vi "getTaskReference.vi"(8 "error in (no error)":errorcluster, 11 "ITaskClassTemplate in":refnum<class "ITaskClassTemplate.lvclass">) -> (0 "error out":errorcluster, 2 "taskRef":refnum<vi>, 3 "ITaskClassTemplate out":refnum<class "ITaskClassTemplate.lvclass">)   [LabVIEW 2023, in "ITaskClassTemplate.lvclass"]
doc: "Returns the VI reference related to the task to handle.\n_____________________________________\nTLC Daemon 1.0.0.6\nCopyright (c) 2026 Andrea Cadei"
uses:
  ITaskClassTemplate.lvclass
  ITaskClassTemplate.lvclass/ITaskClassTemplate.ctl
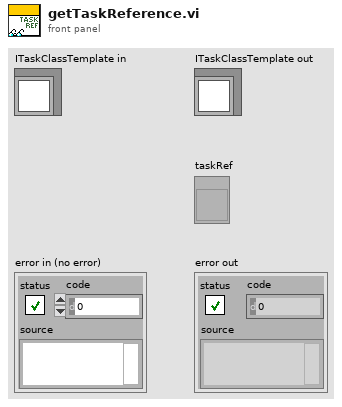
[diagram p1: front panel]
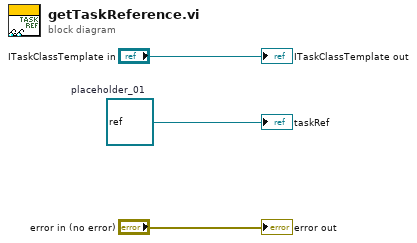
[diagram p0: block diagram]
diagram:
  w1 = refnum<class> refnum  # placeholder_01
  "error out" <- "error in (no error)"
  "ITaskClassTemplate out" <- "ITaskClassTemplate in"
  "taskRef" <- w1
